vi "save_motor_positions.vi"(6 "Echo Mode":i32, 7 "file path (use dialog)":path, 8 "error in":errorcluster={"status"=FALSE, "code"=1073676294, "source"="VISA Read in write_read.vi"}, 11 "ComPort":refnum<visa-resource-name>="COM11") -> (0 "error out":errorcluster={"status"=FALSE, "code"=1073676294, "source"="VISA Read in write_read.vi"}, 2 "Positions":string, 3 "VISA ressource out":refnum<visa-resource-name>)   [LabVIEW 2018]
uses:
  MCode_LV_86/Set Parameter.ctl
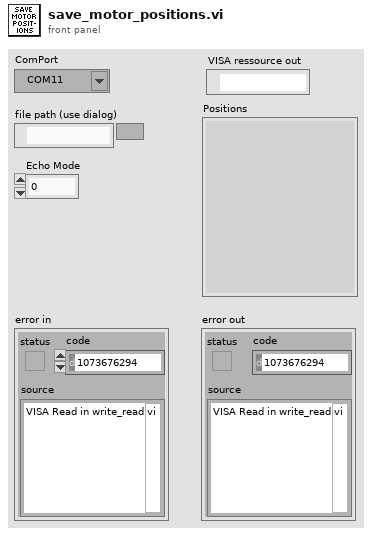
[diagram p1: front panel]
types:
  T1 = enum16{"open", "replace", "create", "open or create", "replace or create", "replace or create with confirmation"}
  T2 = typedef "Set Parameter.ctl" = enum16{"Acceleration (A)", "Baud Rate (BD)", "Counter 1 (C1)", "Counter 2 (C2)", "Control C Software Reset (CE)", "Check Sum Enable (CK)", "Clock Mode (CM)", "Clock Mode Ratio (CR)", "Clock Mode Out Step Width (CW)", "Deceleration (D)", "Digital Filtering, Input 1 (D1)", "Digital Filtering, Input 2 (D2)", "Digital Filtering, Input 3 (D3)", "Digital Filtering, Input 4 (D4)", "Digital Filtering, Input 5 (D5)", "Digital Filtering, Input 9 (D9)", "Digital Filtering, Input 10 (D10)", "Digital Filtering, Input 11 (D11)", "Digital Filtering, Input 12 (D12)", "Deadband (DB)", "Decrement Variable (DC)", "Enable/Disable Drive (DE)", "Device Name (DN)", "End Program Execution (E)", "Encoder Function Enable (EE)", "Error Flag (EF)", "Encoder Lines (EL)", "Echo Mode (EM)", "Error Value (ER)", "Escape (ES)", "Execute Program at Address (EX)", "Firmware Version (VR)", "Hold (H)", "Hold Current (HC)", "Hold Current Delay Time (HI)", "Home to Encoder Index (HM)", "Home to Home Switch (HT)", "Increment Variable (IC)", "Initialize Parameters to NVM (IP)", "Input into Variable (IV)", "Jog Enable (JE)", "Limit Stop Mode (LM)", "Move Absolute (MA)", "Move Relative (MR)", "MicroStepping Select (MS)", "Motor Settling Delay Time (MT)", "Moving [Flag] (MV)", "Output 1 (O1)", "Output 2 (O2)", "Output 3 (O3)", "Output 4 (O4)", "Output 9 (O9)", "Output 10 (O10)", "Output 11 (O11)", "Output 12 (O12)", "Output High Byte (9-12) (OH)", "Output Low Byte (1-4) (OL)", "Output Total (1-4 and 9-12) (OT)", "Position (P)", "Position Maintenance (PM)", "Party Mode (PY)", "Register 1 (R1)", "Register 2 (R2)", "Register 3 (R3)", "Register 4 (R4)", "Reset Error(\\03)", "Run Current (RC)", "Stall Factor (SF)", "Slew (SL)", "Stall Mode Set (SM)", "Upgrade Firmware (UG)", "Velocity Initial (VI)", "Velocity Maximum (VM)", "Current1 (I1)", "Current2 (I2)", "Current3 (I3)", "Current4 (I4)", "Current5 (I5)", "Current6 (I6)", "Save (S)"}
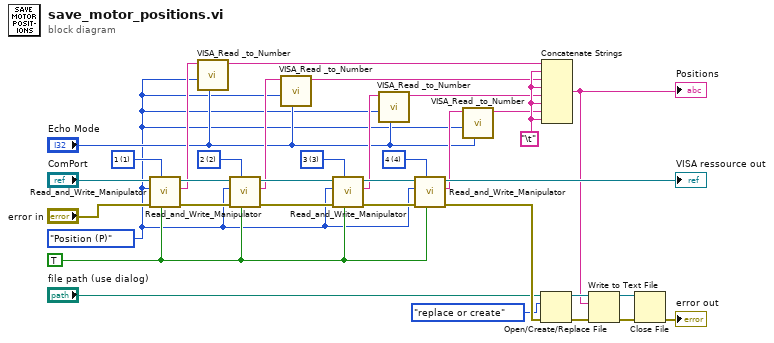
[diagram p0: block diagram]
diagram:
  w21 = "\t"
  w25 = u16 4 items=["none", "1", "2", "3", "4", "all"] ("Motor")
  w7 = u16 3 items=["none", "1", "2", "3", "4", "all"] ("Motor")
  w26 = u16 2 items=["none", "1", "2", "3", "4", "all"] ("Motor")
  w27 = u16 1 items=["none", "1", "2", "3", "4", "all"] ("Motor")
  w28 = TRUE
  w1 = Set_Parameter."Position (P)" ("Command")
  n1 = call "Read_and_Write_Manipulator.vi"("Print?"=w28, "Motor"=w27, "error in (no error)"="error in", "Command"=w1, "VISA resource name"="ComPort") -> ("error out"=w34:errorcluster, "Answer"=w11:string, "VISA ressource out"=w31:refnum<visa-resource-name>)  [unwired: 2 in, 2 out]
  n2 = call "VISA_Read _to_Number.vi"("Echo Mode"="Echo Mode", "Command"=w1, "Answer Buffer"=w11) -> ("number (string)"=w10:string)  [unwired: 7 in, 1 out]
  n3 = call "Read_and_Write_Manipulator.vi"("Print?"=w28, "Motor"=w26, "error in (no error)"=w34, "Command"=w1, "VISA resource name"=w31) -> ("error out"=w33:errorcluster, "Answer"=w9:string, "VISA ressource out"=w30:refnum<visa-resource-name>)  [unwired: 2 in, 2 out]
  n4 = call "VISA_Read _to_Number.vi"("Echo Mode"="Echo Mode", "Command"=w1, "Answer Buffer"=w9) -> ("number (string)"=w8:string)  [unwired: 7 in, 1 out]
  n5 = call "Read_and_Write_Manipulator.vi"("Print?"=w28, "Motor"=w7, "error in (no error)"=w33, "Command"=w1, "VISA resource name"=w30) -> ("error out"=w32:errorcluster, "Answer"=w6:string, "VISA ressource out"=w29:refnum<visa-resource-name>)  [unwired: 2 in, 2 out]
  n6 = call "VISA_Read _to_Number.vi"("Echo Mode"="Echo Mode", "Command"=w1, "Answer Buffer"=w6) -> ("number (string)"=w5:string)  [unwired: 7 in, 1 out]
  n7 = call "Read_and_Write_Manipulator.vi"("Print?"=w28, "Motor"=w25, "error in (no error)"=w32, "Command"=w1, "VISA resource name"=w29) -> ("error out"=w19:errorcluster, "Answer"=w4:string, "VISA ressource out"=→"VISA ressource out":refnum<visa-resource-name>)  [unwired: 2 in, 2 out]
  n8 = call "VISA_Read _to_Number.vi"("Echo Mode"="Echo Mode", "Command"=w1, "Answer Buffer"=w4) -> ("number (string)"=w3:string)  [unwired: 7 in, 1 out]
  n9 = Open/Create/Replace File(file path (use dialog)="file path (use dialog)", error in=w19, operation (0:open)=T1."replace or create") -> (refnum out=w20:refnum<file>, error out=w18:errorcluster)  [unwired: 3 in, 1 out]
  n10 = Concatenate Strings(w10, w21, w8, w21, w5, w21, w3, w21) -> (w17:string)
  "Positions" <- w17
  n11 = Write to Text File(file (use dialog)=w20, text=w17, error in=w18) -> (refnum out=w16:refnum<file>, error out=w15:errorcluster)  [unwired: 1 in, 1 out]
  n12 = Close File(refnum=w16, error in=w15) -> (error out=→"error out":errorcluster)  [unwired: 1 out]
